vi "Get Connected IP.vi"(8 "error in (no error)":errorcluster, 10 "IP Address":string, 11 "Test in":refnum<class "Test.lvclass">) -> (0 "error out":errorcluster, 3 "Test out":refnum<class "Test.lvclass">)   [LabVIEW 2019, in "Test.lvlib" / "Test.lvclass"]
uses:
  Test.lvclass
  Test.lvclass/Test.ctl
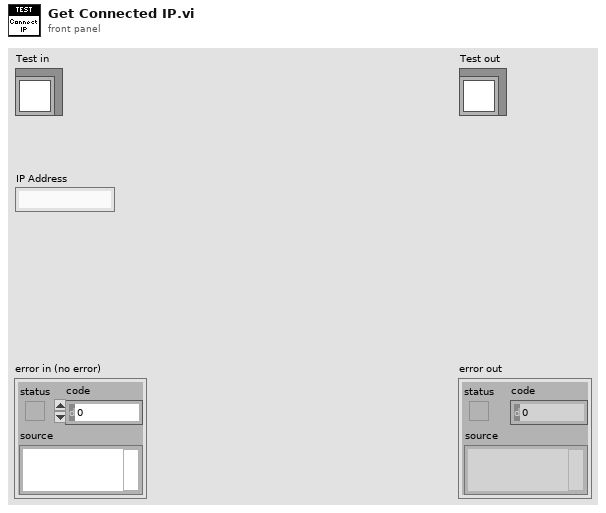
[diagram p1: front panel]
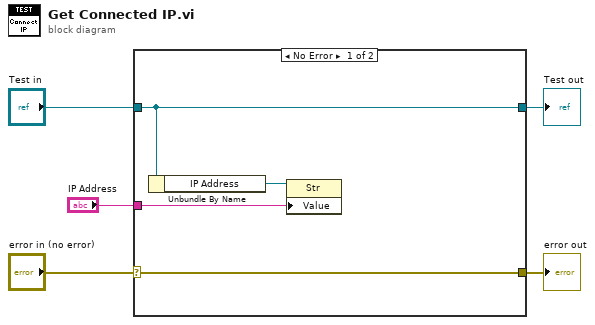
[diagram p0: block diagram]
diagram:
  n1 = case shown="No Error" "error in (no error)" {
    selector: "error in (no error)" -> [w6 w11]
    tunnel: [w6 w11] -> w4
    tunnel: [w9 w10] -> w2
    tunnel: "Test in" -> [w9 w10]
    tunnel: "IP Address" -> [w7 _]
    frame No Error {
      n2 = Unbundle By Name(w9) -> ("IP Address"=w8:refnum<vi>)
      n3 = property class="Str"(reference=w8, "Value"=w7) -> ()  [unwired: 1 in, 2 out]
    }
    frame Error {
    }
  }
  "error out" <- w4
  "Test out" <- w2
